vi "SmartSEM Remote API set string.vi"(5 "Wait (ms)":u32, 7 "Iterations":u32=3, 8 "error in":errorcluster, 9 "vValue":string, 10 "lpszParam":string, 11 "ActiveX Container":refnum<k7>(container)) -> (0 "error out":errorcluster, 3 "reference out":refnum<k7>)   [LabVIEW 2018]
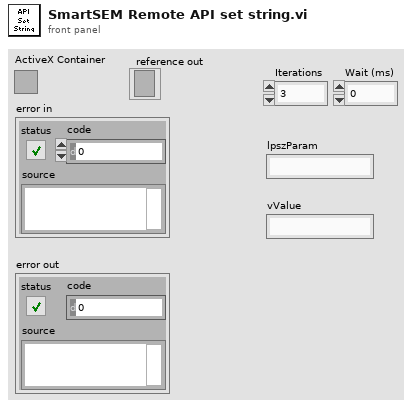
[diagram p1: front panel]
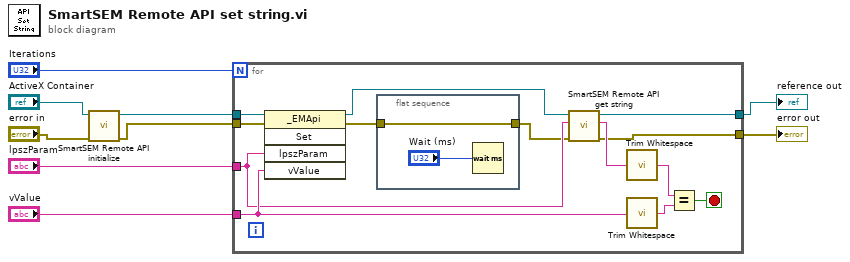
[diagram p0: block diagram]
diagram:
  n1 = call "SmartSEM Remote API initialize.vi"("error in"="error in", "ActiveX Container"="ActiveX Container") -> ("error out"=w4:errorcluster, "reference out"=w3:refnum<k7>)  [unwired: 8 in]
  n2 = for {
    N: "Iterations" -> [_]
    tunnel: w3 -> [w22]
    tunnel: w4 -> [w21]
    tunnel: [w12] -> w5
    tunnel: [w11] -> w6
    tunnel: "vValue" -> [w18]
    tunnel: "lpszParam" -> [w14]
    stop <- w19 stop-if-true
    n3 = invoke class="_EMApi" method="Set"(reference=w22, error in=w21, "lpszParam"=w14, "vValue"=w18) -> (reference out=w15:refnum<k7>, error out=w16:errorcluster)  [unwired: 1 in, 3 out]
    n4 = flat-sequence {
      tunnel: [w24] -> w10
      tunnel: w16 -> [w24]
      frame #0 {
        n5 = Wait (ms)(milliseconds to wait="Wait (ms)") -> ()  [unwired: 1 out]
      }
    }
    n6 = call "SmartSEM Remote API get string.vi"("error in"=w10, "lpszParam"=w14, "ActiveX Container"=w15) -> ("error out"=w11:errorcluster, "data"=w13:string, "reference out"=w12:refnum<k7>)  [unwired: 6 in]
    n7 = call <vilib>:"Trim Whitespace.vi"("string"=w13) -> ("trimmed string"=w20:string)  [unwired: 1 in]
    n8 = call <vilib>:"Trim Whitespace.vi"("string"=w18) -> ("trimmed string"=w17:string)  [unwired: 1 in]
    n9 = Equal?(x=w20, y=w17) -> (x = y?=w19:bool)
  }
  "error out" <- w6
  "reference out" <- w5
